vi "SetMode1.vi"() -> (0 "output cluster":T1 {"EXTclk" format="%x"; "Restart" format="%x"; "AutoInkrement" format="%x"; "sub1" format="%x"; "Sleep" format="%x"; "sub2" format="%x"; "sub3" format="%x"; "Allcall" format="%x"})   [LabVIEW 2022 SP3, in "PCA9685.lvlib" / "PCA.lvclass"]
uses:
  PCA.lvclass
  typedefs/Mode1.ctl
  PCA.lvclass/PCA.ctl
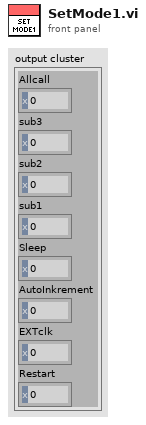
[diagram p1: front panel]
types:
  T1 = typedef "PCA9685.lvlib/PCA.lvclass/Mode1.ctl" = cluster{"Allcall":u8, "sub3":u8, "sub2":u8, "Sleep":u8, "sub1":u8, "AutoInkrement":u8, "Restart":u8, "EXTclk":u8}
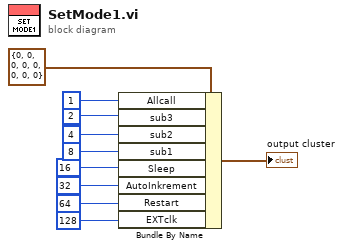
[diagram p0: block diagram]
diagram:
  n1 = Bundle By Name(cluster=T1 {"Allcall"=0, "sub3"=0, "sub2"=0, "Sleep"=0, "sub1"=0, "AutoInkrement"=0, "Restart"=0, "EXTclk"=0} ("Mode1"), "Allcall"=u8 1, "sub3"=u8 2 ("Allcall"), "sub2"=u8 4 ("Allcall"), "sub1"=u8 8 ("Allcall"), "Sleep"=u8 16 ("Allcall"), "AutoInkrement"=u8 32 ("Allcall"), "Restart"=u8 64 ("Allcall"), "EXTclk"=u8 128 ("Allcall")) -> (→"output cluster":T1)
